vi "Generate Packages List.vi"(8 "error in (no error)":errorcluster, 10 "Repos":refnum<class "Repo.lvclass">[](array[class]), 11 "LabVIEW Web Service":refnum<class "Web Service.lvclass">) -> (0 "error out":errorcluster, 3 "LabVIEW Web Service out":refnum<class "Web Service.lvclass">)   [LabVIEW 2020, in "Packages.lvlib"]
uses:
  Packages.lvlib
  Repo_class/Repo.lvclass
  <vilib>/wsapi/Web Service.lvclass
  Repo_class/Repo.lvclass/Repo.ctl
  Package_class/Package.lvclass/Package.ctl
  Package Version_class/Package Version.lvclass/Package Version.ctl
  Repo_class/Read Packages.vi
  Package_class/Read DisplayName.vi
  Package_class/Read Versions.vi
  Package_class/Read Name.vi
  Package Version_class/Read Vendor.vi
  Package_class/Package.lvclass
  Package Version_class/Package Version.lvclass
  WSsupport/WSsupport.lvlib
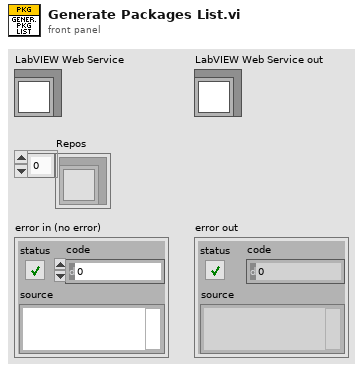
[diagram p1: front panel]
types:
  T1 = enum16{"open", "replace", "create", "open or create", "replace or create", "replace or create with confirmation"}
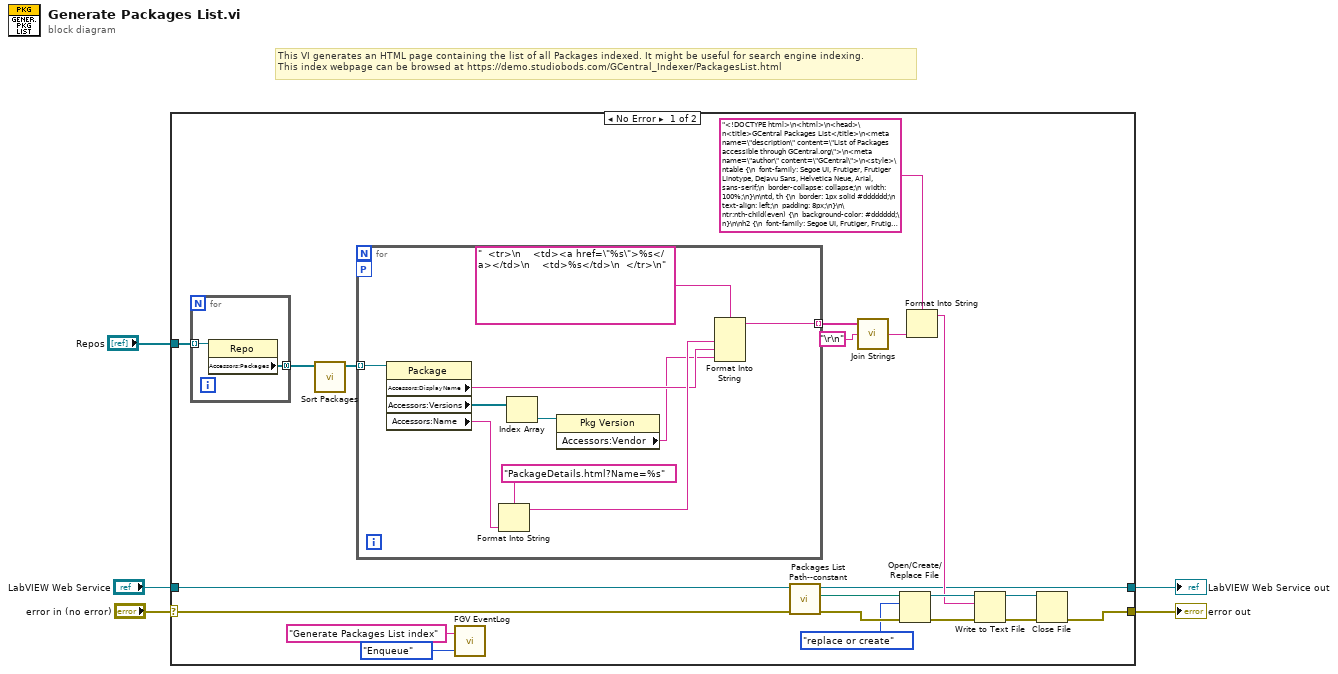
[diagram p0: block diagram]
diagram:
  # "This VI generates an HTML page containing the list of all Packages indexed. It might be useful for search engine indexing.\nThis index webpage can be browsed at https://demo.studiobods.com/GCentral_Indexer/PackagesList.html"
  n1 = case shown="No Error" "error in (no error)" {
    selector: "error in (no error)" -> [w23 w40]
    tunnel: "Repos" -> [w26 _]
    tunnel: [w13 w40] -> w3
    tunnel: "LabVIEW Web Service" -> [w9 w39]
    tunnel: [w8 w39] -> w1
    frame No Error {
      n2 = for {
        tunnel: [w38] -> w25 mode=concatenating
        tunnel: w26 -> [w37] mode=indexing
        n3 = property class="Repo"(reference=w37) -> ("Accessors:Packages"=w38:refnum<class "Package.lvclass">[])  [unwired: 1 in, 2 out]
      }
      n4 = call "Sort Packages.vi"("Packages"=w25) -> ("Sorted Packages"=w24:refnum<class "Package.lvclass">[])  [unwired: 10 in]
      n5 = for {
        tunnel: w24 -> [w36] mode=indexing
        tunnel: [w27] -> w22 mode=indexing
        workers-P: _ -> [_]
        n6 = property class="Package"(reference=w36) -> ("Accessors:DisplayName"=w30:string, "Accessors:Versions"=w33:refnum<class "Package Version.lvclass">[], "Accessors:Name"=w34:string)  [unwired: 1 in, 2 out]
        n7 = Format Into String(format string="PackageDetails.html?Name=%s", w34) -> (resulting string=w31:string)  [unwired: 2 in, 1 out]
        n8 = Index Array(array=w33) -> (element=w32:refnum<class "Package Version.lvclass">)  [unwired: 1 in]
        n9 = property class="Pkg Version"(reference=w32) -> ("Accessors:Vendor"=w29:string)  [unwired: 1 in, 2 out]
        n10 = Format Into String(format string="  <tr>\n    <td><a href=\"%s\">%s</a></td>\n    <td>%s</td>\n  </tr>\n", w31, w30, w29) -> (resulting string=w27:string)  [unwired: 2 in, 1 out]
      }
      n11 = call "FGV EventLog.vi"("Action"=enum16{"Reset", "Enqueue", "Dequeue"}."Enqueue", "String to log"="Generate Packages List index") -> ()  [unwired: 1 in, 1 out]
      n12 = call "Packages List Path--constant.vi"("error in (no error)"=w23, "LabVIEW Web Service"=w9) -> ("error out"=w18:errorcluster, "Packages index path"=w16:path, "LabVIEW Web Service out"=w8:refnum<class "Web Service.lvclass">)  [unwired: 7 in]
      n13 = call <vilib>:"Join Strings.vi"("Separator (,)"="\r\n", "Strings In"=w22) -> ("String"=w20:string)  [unwired: 1 in]
      n14 = Open/Create/Replace File(file path (use dialog)=w16, error in=w18, operation (0:open)=T1."replace or create") -> (refnum out=w12:refnum<file>, error out=w17:errorcluster)  [unwired: 3 in, 1 out]
      n15 = Format Into String(format string="<!DOCTYPE html>\n<html>\n<head>\n<title>GCentral Packages List</title>\n<meta name=\"description\" content=\"List of Packages accessible through GCentral.org\">\n<meta name=\"author\" content=\"GCentral\">\n<style>\ntable {\n  font-family: Segoe UI, Frutiger, Frutiger Linotype, Dejavu Sans, Helvetica Neue, Arial, sans-serif;\n  border-collapse: collapse;\n  width: 100%;\n}\n\ntd, th {\n  border: 1px solid #dddddd;\n  text-align: left;\n  padding: 8px;\n}\n\ntr:nth-child(even) {\n  background-color: #dddddd;\n}\n\nh2 {\n  font-family: Segoe UI, Frutiger, Frutiger Linotype, Dejavu Sans, Helvetica Neue, Arial, sans-serif;\n  text-align:center;\n}\n\n.center {\n  display: block;\n  margin-left: auto;\n  margin-right: auto;\n  width: 50%;\n}\n</style>\n</head>\n<body>\n\n<picture>\n  <img src=\"https://demo.studiobods.com/GCentral_Indexer/images/logo.png\" alt=\"Logo\" style=\"width:auto;\" class=\"center\">\n</picture>\n\n<h2>GCentral Packages List</h2>\n\n<table align=\"center\">\n  <tr>\n    <th>Package</th>\n    <th>Vendor</th>\n  </tr>%s\n</table>\n\n</body>\n</html>\n", w20) -> (resulting string=w10:string)  [unwired: 2 in, 1 out]
      n16 = Write to Text File(file (use dialog)=w12, text=w10, error in=w17) -> (refnum out=w11:refnum<file>, error out=w14:errorcluster)  [unwired: 1 in, 1 out]
      n17 = Close File(refnum=w11, error in=w14) -> (error out=w13:errorcluster)  [unwired: 1 out]
    }
    frame Error {
    }
  }
  "error out" <- w3
  "LabVIEW Web Service out" <- w1
